vi "Read X.vi"(8 "error in (no error)":errorcluster, 11 "Class in":refnum<class "Class with PropertyNode.lvclass">) -> (0 "error out":errorcluster, 2 "X":dbl, 3 "Class out":refnum<class "Class with PropertyNode.lvclass">)   [LabVIEW 2021, in "Class with PropertyNode.lvclass"]
uses:
  Class with PropertyNode.lvclass
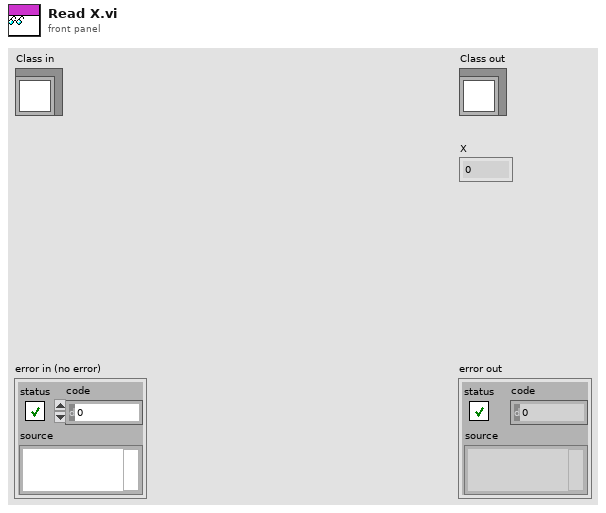
[diagram p1: front panel]
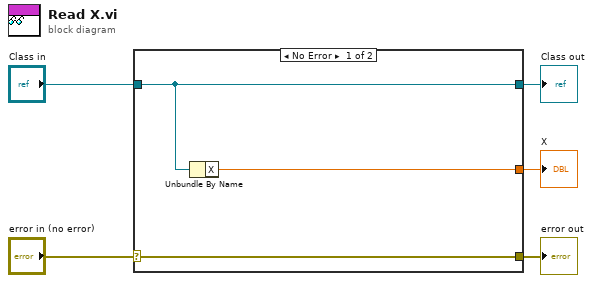
[diagram p0: block diagram]
diagram:
  n1 = case shown="No Error" "error in (no error)" {
    selector: "error in (no error)" -> [w8 w9]
    tunnel: [w8 w9] -> w4
    tunnel: [w7 w10] -> w2
    tunnel: "Class in" -> [w7 w10]
    tunnel: [w6 _] -> w1
    frame No Error {
      n2 = Unbundle By Name(w7) -> ("X"=w6:dbl)
    }
    frame Error {
    }
  }
  "error out" <- w4
  "Class out" <- w2
  "X" <- w1
